vi "SymMatrix EigenVectors and Values.vi"(0 "Input Matrix":T2, 1 "output option":T1=1 items=["Eigenvalues", "Eigenvalues & Vectors"]) -> (2 "Eigenvalue":dbl[](array[numeric]), 3 "Eigenvector":T2, 4 "error":i32)   [LabVIEW 2017, in "NI_AALBase.lvlib"]
uses:
  NI_AALBase.lvlib
  RealMatrix.ctl
  Eigenvalue and Vectors Output Option.ctl
  lvanlys.dll
  NI_Matrix.lvlib
  NI_AALPro.lvlib
panel:
  # "SymMatrix EigenVectors and Values"
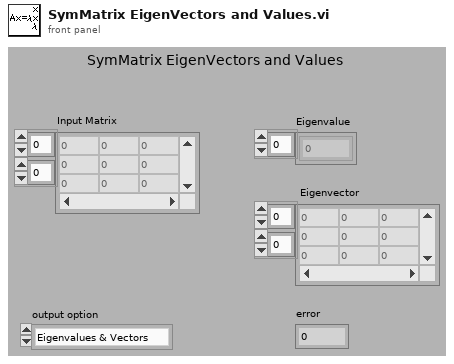
[diagram p1: front panel]
types:
  T1 = typedef "NI_AALPro.lvlib/Eigenvalue and Vectors Output Option.ctl" = i32
  T2 = typedef "NI_Matrix.lvlib/RealMatrix.ctl" = dbl[][]
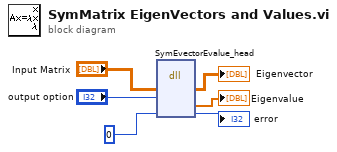
[diagram p0: block diagram]
diagram:
  n1 = dll-call lib="C:/Program Files/National Instruments/LabVIEW 2017/resource/lvanlys.*" fn="SymEvectorEvalue_head"("Input Matrix"="Input Matrix", "output option"="output option", 0) -> ("Input Matrix"=→"Eigenvector":T2, "Eigenvalue"=→"Eigenvalue":dbl[], →"error":i32)  [unwired: 6 in, 2 out]
